vi "build_using.vi"(10 "scan_pars_refnum":refnum<vi>, 11 "build_using":T1(ring)) -> ()   [LabVIEW 2013, in "tools.lvlib"]
uses:
  tools.lvlib
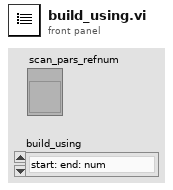
[diagram p1: front panel]
types:
  T1 = enum16{"start: end: num", "start: step: end", "start: step: num"}
  T2 = enum8{"Enabled", "Disabled", "Disabled and Grayed Out"}
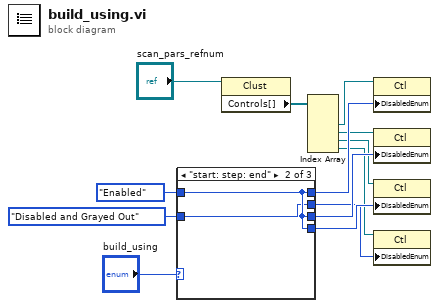
[diagram p0: block diagram]
diagram:
  n1 = case shown="\"start: step: end\"" "build_using" {
    tunnel: T2."Enabled" ("Disabled") -> [w15 w17 w19]
    tunnel: [w15 w17 w18] -> w3
    tunnel: [w15 w17 w19] -> w7
    tunnel: [w14 w17 w19] -> w5
    tunnel: [w15 w16 w19] -> w1
    tunnel: T2."Disabled and Grayed Out" ("Disabled") -> [w14 w16 w18]
    frame "start: end: num", Default {
    }
    frame "start: step: end" {
    }
    frame "start: step: num" {
    }
  }
  n2 = property class="Clust"(reference="scan_pars_refnum") -> ("Controls[]"=w10:refnum<vi>[])  [unwired: 1 in, 2 out]
  n3 = Index Array(array=w10) -> (element #2=w9:refnum<vi>, element #3=w6:refnum<vi>, element #4=w4:refnum<vi>, element #5=w2:refnum<vi>)  [unwired: 5 in, 1 out]
  n4 = property class="Ctl"(reference=w9, "DisabledEnum"=w7) -> ()  [unwired: 1 in, 2 out]
  n5 = property class="Ctl"(reference=w6, "DisabledEnum"=w5) -> ()  [unwired: 1 in, 2 out]
  n6 = property class="Ctl"(reference=w4, "DisabledEnum"=w3) -> ()  [unwired: 1 in, 2 out]
  n7 = property class="Ctl"(reference=w2, "DisabledEnum"=w1) -> ()  [unwired: 1 in, 2 out]
